vi "shutdown_ppms.vi"   [LabVIEW 2019]
uses:
  Global/Global Variables/Data_Display_global.vi
types:
  T1 = typedef "P9P14-TCluster.ctl" = cluster{"Setpoint":dbl, "Rate":dbl, "Chanel 1":dbl, "Approach":u16, "Set":bool, "Temperature\nStatus":i32, "Autoshutdown":bool}
  T2 = typedef "P9P14-TCluster-Control.ctl" = cluster{"Setpoint":dbl, "Rate":dbl, "Approach":u16, "Set":bool, "Autoshutdown":bool}
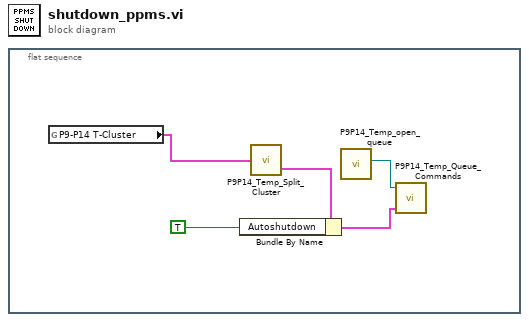
[diagram p0: block diagram]
diagram:
  n1 = flat-sequence {
    frame #0 {
      n2 = global read "Data_Display_global.vi" "P9-P14 T-Cluster"() -> (w4:T1)
      n3 = call "P9P14_Temp_Split_Cluster.vi"("P9-P14 T-Cluster"=w4) -> ("P9-P14 T-Cluster -Control"=w3:T2)  [unwired: 1 out]
      n4 = Bundle By Name(cluster=w3, "Autoshutdown"=TRUE) -> (w1:T2)
      n5 = call "P9P14_Temp_open_queue.vi"() -> ("queue out"=w5:refnum<queue>)  [unwired: 10 in, 1 out]
      n6 = call "P9P14_Temp_Queue_Commands.vi"("P9-P14 T-Cluster -Control"=w1, "Queue"=w5) -> ()  [unwired: 1 in, 1 out]
    }
  }
